vi "Set Blob Properties.vi"(6 "Header name-value pairs":T1[](array[typedef]), 8 "error in (no error)":errorcluster, 9 "Blob":string, 10 "Container":string, 11 "Azure Session in":refnum<class "Session.lvclass">) -> (0 "error out":errorcluster, 3 "Azure Session out":refnum<class "Session.lvclass">)   [LabVIEW 2015, in "NI_Azure_Blob.lvlib"]
doc: "Sets system properties defined for an existing blob."
uses:
  NI_Azure_Blob.lvlib
  Core/Session/Session.lvclass
  Core/Name Value Pair.ctl
  Core/Session/Session.lvclass/Session.ctl
  Core/Session/Write Request Headers.vi
  Core/Session/Write Request Parameters.vi
  Core/Session/Write URL Suffix.vi
  Core/Session/Write HTTP Verb.vi
  Core/NI_Azure_Core.lvlib
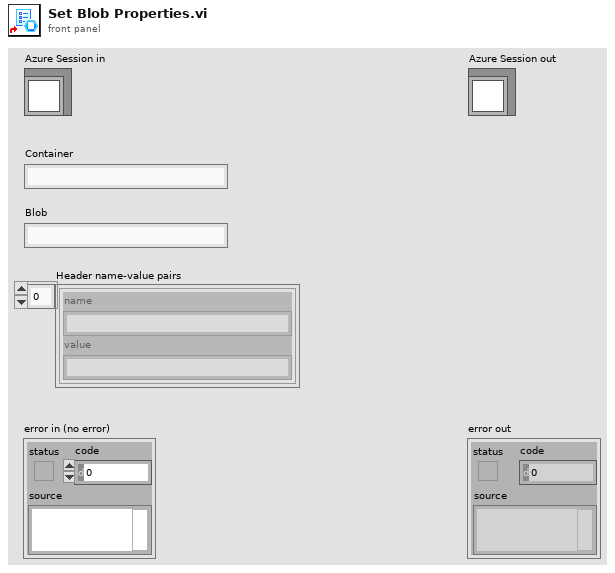
[diagram p1: front panel]
types:
  T1 = typedef "NI_Azure_Core.lvlib/Name Value Pair.ctl" = cluster{"name":string, "value":string}
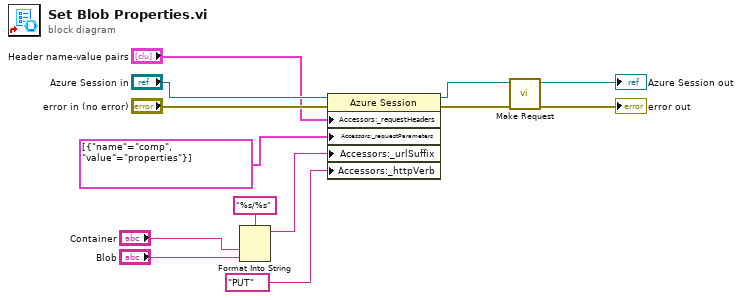
[diagram p0: block diagram]
diagram:
  n1 = Format Into String(format string="%s/%s", "Container", "Blob") -> (resulting string=w2:string)  [unwired: 2 in, 1 out]
  n2 = property class="Azure Session"(reference="Azure Session in", error in="error in (no error)", "Accessors:_requestHeaders"="Header name-value pairs", "Accessors:_requestParameters"=T1[] [{"name"="comp", "value"="properties"}] ("request parameters"), "Accessors:_urlSuffix"=w2, "Accessors:_httpVerb"="PUT" ("HTTP-Verb")) -> (reference out=w5:refnum<class "Session.lvclass">, error out=w7:errorcluster)
  n3 = call "Make Request.vi"("error in (no error)"=w7, "Session in"=w5) -> ("error out"=→"error out":errorcluster, "Session out"=→"Azure Session out":refnum<class "Session.lvclass">)  [unwired: 7 in, 1 out]
